vi "_API_BINANCE_POST_USDT_FEATURES_changeIsolated.vi"(0 "BinanceAPI in":refnum<class "BinanceAPI_.lvclass">, 5 "Change Margin Type":T1={"symbol (BTCUSDT)"="", "recvWindow"=5000, "marginTypa"=enum."NaN"}, 11 "error in (no error)":errorcluster) -> (4 "BinanceAPI out":refnum<class "BinanceAPI_.lvclass">, 14 "Body":string, 15 "error out":errorcluster)   [LabVIEW 2022 SP3, in "BinanceAPI_.lvclass"]
doc: "https://binance-docs.github.io/apidocs/futures/en/#change-margin-type-trade"
uses:
  BinanceAPI_.lvclass
  BinanceAPI_.lvclass/BinanceAPI_.ctl
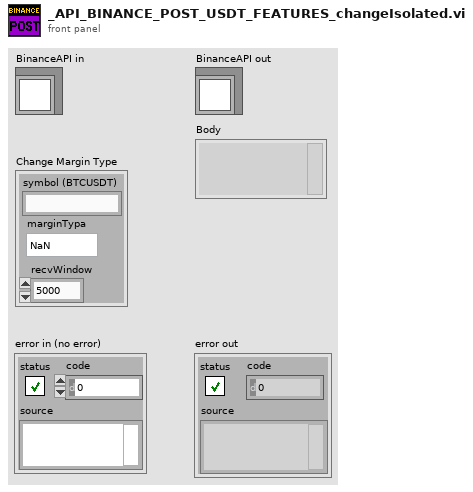
[diagram p1: front panel]
types:
  T1 = cluster{"symbol (BTCUSDT)":string, "recvWindow":i32, "marginTypa":enum16{"NaN", "CROSSED", "ISOLATED"}}
  T2 = enum16{"SPOT", "USDT_FUTURES", "COIN_FUTURES", "VANILLA"}
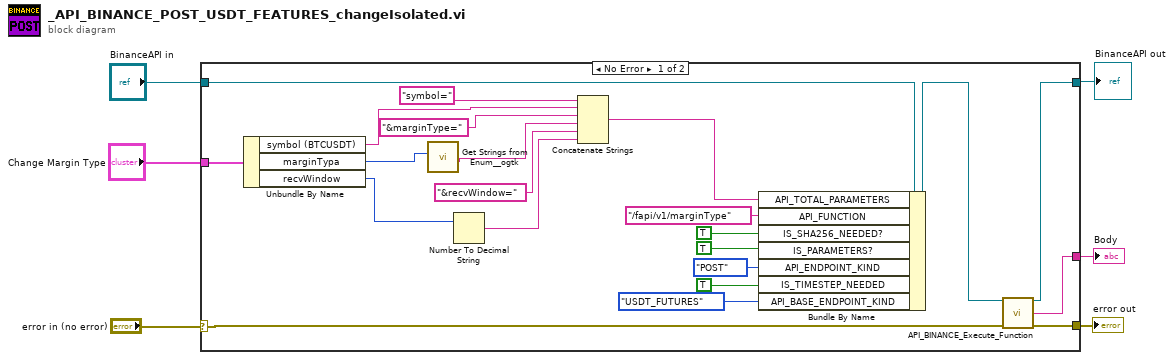
[diagram p0: block diagram]
diagram:
  n1 = case shown="No Error" "error in (no error)" {
    selector: "error in (no error)" -> [w19 w30]
    tunnel: [w15 w30] -> w5
    tunnel: [w16 w29] -> w1
    tunnel: "BinanceAPI in" -> [w20 w29]
    tunnel: "Change Margin Type" -> [w25 _]
    tunnel: [w7 _] -> w3
    frame No Error {
      n2 = Unbundle By Name(w25) -> ("symbol (BTCUSDT)"=w22:string, "marginTypa"=w9:enum16{"NaN", "CROSSED", "ISOLATED"}, "recvWindow"=w13:i32)
      n3 = call <userlib>:"Get Strings from Enum__ogtk.vi"("Enum"=w9) -> ("String Value"=w8:string)  [unwired: 7 in, 3 out]
      n4 = Number To Decimal String(number=w13) -> (decimal integer string=w10:string)  [unwired: 1 in]
      n5 = Concatenate Strings("symbol=" ("Symbol"), w22, "&marginType=" ("Symbol"), w8, "&recvWindow=" ("Symbol"), w10) -> (w24:string)
      n6 = Bundle By Name(cluster=w20, "API_TOTAL_PARAMETERS"=w24, "API_FUNCTION"="/fapi/v1/marginType", "IS_SHA256_NEEDED?"=TRUE, "IS_PARAMETERS?"=TRUE, "API_ENDPOINT_KIND"=enum16{"POST", "DELETE", "GET", "PUT"}."POST", "IS_TIMESTEP_NEEDED"=TRUE ("IS_PARAMETERS?"), "API_BASE_ENDPOINT_KIND"=T2."USDT_FUTURES") -> (w17:refnum<class "BinanceAPI_.lvclass">)
      n7 = call "API_BINANCE_Execute_Function.vi"("BinanceAPI in"=w17, "error in (no error)"=w19) -> ("BinanceAPI out"=w16:refnum<class "BinanceAPI_.lvclass">, "Body"=w7:string, "error out"=w15:errorcluster)  [unwired: 9 in, 2 out]
    }
    frame Error {
    }
  }
  "error out" <- w5
  "Body" <- w3
  "BinanceAPI out" <- w1
